vi "PNDT - subsampling data reduction.vi"(8 "sub-sampling":T1=1 items=["", "1:1", "2:1", "3:1", "4:1", "5:1", "6:1", "7:1", "8:1", "9:1", "10:1"], 10 "header (1A)":u8=26 format="%.0x", 11 "data set":u16[](array[numeric])) -> (2 "reduced data set":u16[](array[numeric]), 3 "scan length":i32)   [LabVIEW 2026, in "MicroPulse_Driver.lvlib"]
doc: "Decimates data by only retaining maximum peaks and discarding rest of set.\n\n50% = 1 in 2\n66% = 1 in 3\n75% = 1 in 4\n80% = 1 in 5\n90% = 1 in 10\n\n!! USE WITH CARE !!"
uses:
  MicroPulse_Driver.lvlib
  Public/Data/Datatypes/PNDT - subsampling.ctl
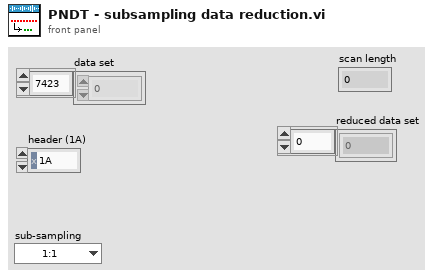
[diagram p1: front panel]
types:
  T1 = typedef "MicroPulse_Driver.lvlib/PNDT - subsampling.ctl" = u16
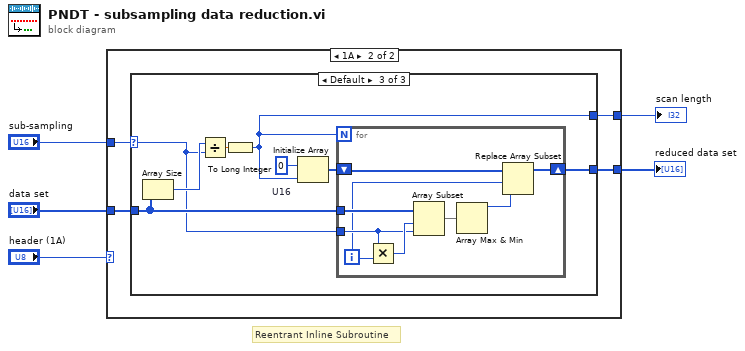
[diagram p0: block diagram]
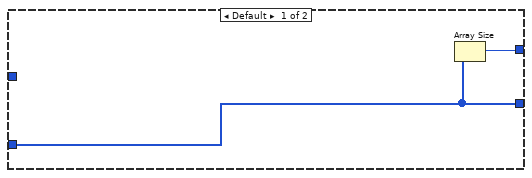
[diagram p2: hidden frame]
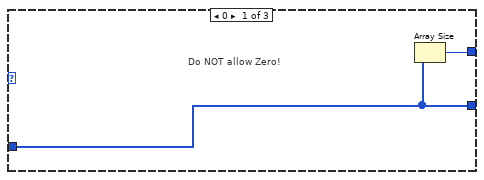
[diagram p3: hidden frame]
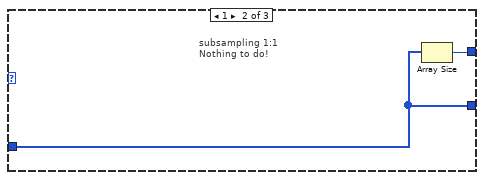
[diagram p4: hidden frame]
diagram:
  # "Reentrant Inline Subroutine"
  n1 = case shown="1A" "header (1A)" {
    tunnel: "data set" -> [w6 w11]
    tunnel: [w6 w10] -> w4
    tunnel: "sub-sampling" -> [_ w9]
    tunnel: [w7 w8] -> w1
    frame Default {
      n2 = Array Size(array=w6) -> (size(s)=w7:i32)
    }
    frame 26 {
      n3 = case shown="Default" w9 {
        selector: w9 -> [_ _ w18]
        tunnel: w11 -> [w12 w15 w20]
        tunnel: [w12 w15 w19] -> w10
        tunnel: [w13 w14 w16] -> w8
        frame 0 {
          # "Do NOT allow Zero!"
          n4 = Array Size(array=w12) -> (size(s)=w13:i32)
        }
        frame 1 {
          # "subsampling 1:1\nNothing to do!"
          n5 = Array Size(array=w15) -> (size(s)=w14:i32)
        }
        frame Default {
          w22 = u16 0  # U16
          n6 = Array Size(array=w20) -> (size(s)=w21:i32)
          n7 = Divide(x=w21, y=w18) -> (x/y=w17:dbl)
          n8 = To Long Integer(number=w17) -> (32bit integer=w16:i32)
          n9 = Initialize Array(w22, w16) -> (w23:u16[])
          n10 = for {
            N: w16 -> [_]
            tunnel: w18 -> [w29]
            shift-right: [w28] -> w19
            shift-left: w23 -> [w27]
            tunnel: w20 -> [w31]
            i -> [w26]
            n11 = Multiply(x=w29, y=w26) -> (x*y=w30:i32)
            n12 = Array Subset(array=w31, index=w30, length=w29) -> (w24:u16[])
            n13 = Array Max & Min(array=w24) -> (max value=w25:u16)  [unwired: 3 out]
            n14 = Replace Array Subset(array=w27, new element=w25, index=w26) -> (w28:u16[])
          }
        }
      }
    }
  }
  "reduced data set" <- w4
  "scan length" <- w1
